vi "VerifyLabVIEWCLI.vi"(8 "Error In":errorcluster) -> (0 "Error Out":errorcluster)   [LabVIEW 2019, in "MicronClient.lvclass"]
uses:
  MicronClient.lvclass
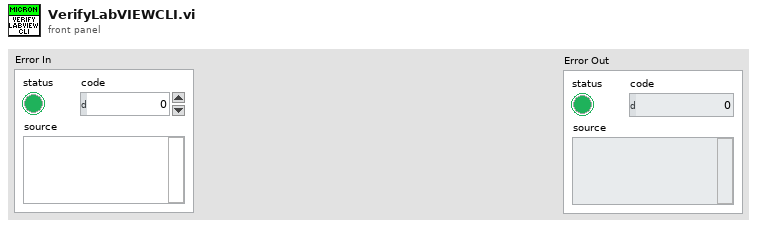
[diagram p1: front panel]
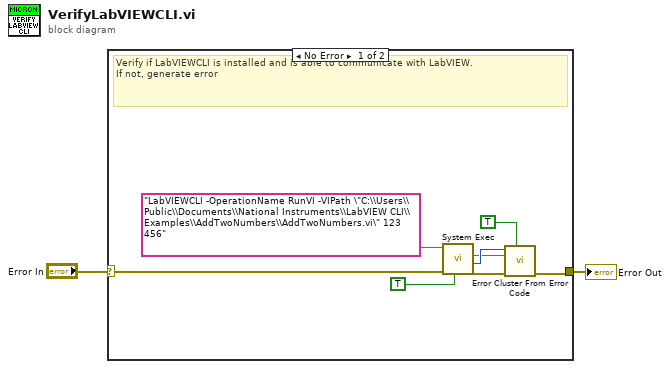
[diagram p0: block diagram]
diagram:
  n1 = case shown="No Error" "Error In" {
    selector: "Error In" -> [w10 w11]
    tunnel: [w5 w11] -> w1
    frame No Error {
      # "Verify if LabVIEWCLI is installed and is able to communicate with LabVIEW. \nIf not, generate error"
      n2 = call <vilib>:"System Exec.vi"("run minimized? (F)"=TRUE, "error in (no error)"=w10, "command line"="LabVIEWCLI -OperationName RunVI -VIPath \"C:\\Users\\Public\\Documents\\National Instruments\\LabVIEW CLI\\Examples\\AddTwoNumbers\\AddTwoNumbers.vi\" 123 456") -> ("error out"=w9:errorcluster, "return code"=w8:i32, "standard error"=w7:string)  [unwired: 5 in, 1 out]
      n3 = call <vilib>:"Error Cluster From Error Code.vi"("show call chain? (False)"=TRUE, "error in (no error)"=w9, "error message (\"\")"=w7, "error code (0)"=w8) -> ("error out"=w5:errorcluster)  [unwired: 5 in]
    }
    frame Error {
    }
  }
  "Error Out" <- w1
